vi "Event Based Structures.vi"() -> ()   [LabVIEW 2011]
panel:
  in  "Boolean":bool
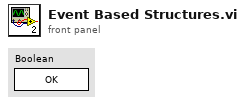
[diagram p1: front panel]
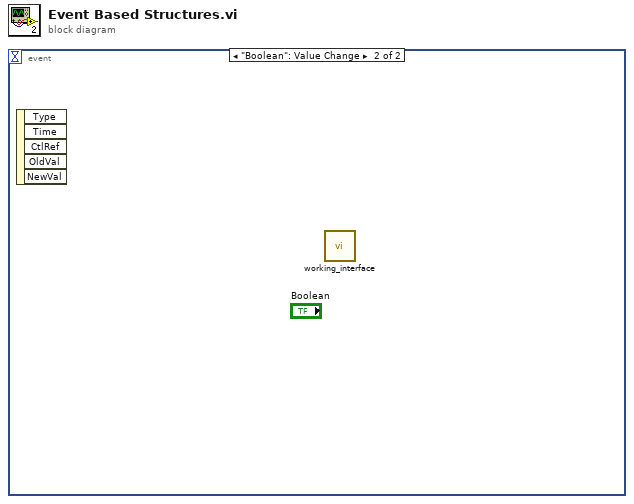
[diagram p0: block diagram]
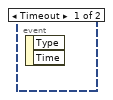
[diagram p2: hidden frame]
diagram:
  n1 = event shown="[1] \"Boolean\": Value Change" {
    selector: _ -> [_ _]
    dyn-events: _ -> [_ _]
    timeout: _ -> [_ _]
    event Timeout {
      n2 = event-data() -> ()  [unwired: 1 in, 2 out]
    }
    event "Boolean": Value Change {
      n3 = event-data() -> ()  [unwired: 1 in, 5 out]
      n4 = call "working_interface.vi"() -> ()  [unwired: 11 in, 1 out]
    }
  }
